vi "Feed-V-Probe-Graph.vi"(6 "Boolesch":bool, 7 "Numerisch":i32, 9 "Array 2":dbl[][](array[numeric]), 10 "Array":dbl[](array[numeric]), 11 "Start fit (% of rec. period)":dbl) -> (3 "Array 3":cluster{dbl[], dbl[]}[](array[cluster]))   [LabVIEW 2024]
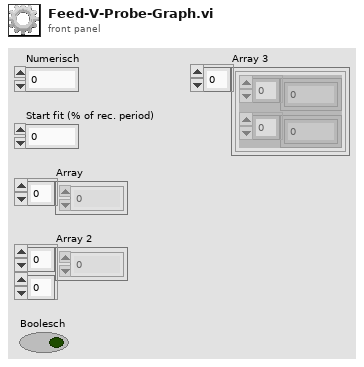
[diagram p1: front panel]
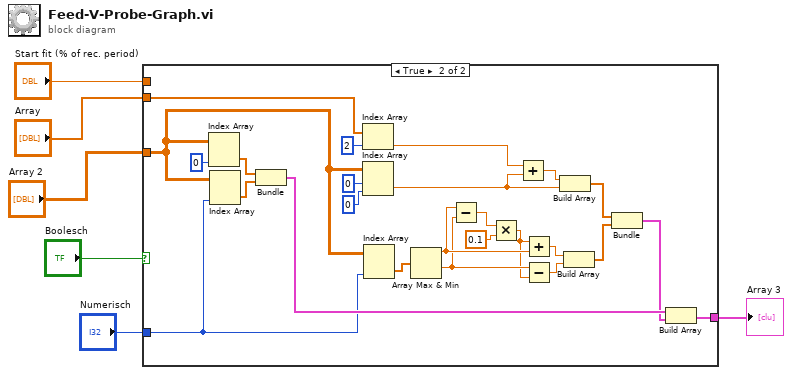
[diagram p0: block diagram]
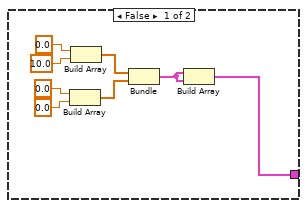
[diagram p2: hidden frame]
diagram:
  n1 = case shown="True" "Boolesch" {
    tunnel: [w7 w19] -> w1
    tunnel: "Array 2" -> [_ w18]
    tunnel: "Array" -> [_ w17]
    tunnel: "Start fit (% of rec. period)" -> [_ _]
    tunnel: "Numerisch" -> [_ w15]
    frame False {
      n2 = Build Array(0.0, 0.0) -> (w9:dbl[])
      n3 = Build Array(0.0, 10.0) -> (w10:dbl[])
      n4 = Bundle(w10, w9) -> (w8:cluster{dbl[], dbl[]})  [unwired: 1 in]
      n5 = Build Array(w8, w8) -> (w7:cluster{dbl[], dbl[]}[])
    }
    frame True {
      n6 = Index Array(array=w18, index (col)=0 ("disabled index (col)")) -> (element=w38:dbl[])  [unwired: 1 in]
      n7 = Index Array(array=w18, index (col)=w15) -> (element=w39:dbl[])  [unwired: 1 in]
      n8 = Bundle("Array 2"=w38, "Array 2"=w39) -> (w36:cluster{"Array 2":dbl[], "Array 2":dbl[]})  [unwired: 1 in]
      n9 = Index Array(array=w17, index=2) -> (element=w21:dbl)
      n10 = Index Array(array=w18, index (row)=0, index (col)=0) -> (element=w22:dbl)
      n11 = Index Array(array=w18, index (col)=w15) -> (element=w34:dbl[])  [unwired: 1 in]
      n12 = Array Max & Min(array=w34) -> (max value=w30:dbl, min value=w29:dbl)  [unwired: 2 out]
      n13 = Subtract(x=w30, y=w29) -> (x-y=w33:dbl)
      n14 = Multiply(x=w33, y=0.1) -> (x*y=w27:dbl)
      n15 = Add(x=w21, y=w22) -> (x+y=w23:dbl)
      n16 = Add(x=w27, y=w30) -> (x+y=w31:dbl)
      n17 = Subtract(x=w29, y=w27) -> (x-y=w28:dbl)
      n18 = Build Array(w23, w22) -> (w20:dbl[])
      n19 = Build Array(w31, w28) -> (w35:dbl[])
      n20 = Bundle(w20, w35) -> (w16:cluster{dbl[], dbl[]})  [unwired: 1 in]
      n21 = Build Array(w36, w16) -> (w19:cluster{"Array 2":dbl[], "Array 2":dbl[]}[])
    }
  }
  "Array 3" <- w1
